vi "Sort 2D String Array - Preview Sorted Array.vi"(7 "Sorted Data Preview":string[][](table)) -> (8 "Output Array":string[][](array[string]), 10 "User Cancelled":bool)   [LabVIEW 2009]
doc: "Sort 2D String Array - Preview Sorted Array.vi\n\n<B>Description:</B>\n\nThis VI enables the user to preview the sorted array and accept or cancel the sort.\n\nThe user can press the Accept Sort button to accept the sorted array as displayed. If the Accept Sort button is pressed, the input array is passed to the Output Array terminal.\n\nThe user can press the Cancel Sort button to cancel the sort. If the Cancel Sort button is pressed, an empty array is passed to the Output Array terminal.\n\n<B>Usage:</B>\n\nWire all required inputs.\n\n<B>Inputs:</B>\n\nSorted Data Preview\n- This is the input 2D array of strings that will be previewed.\n\n<B>Outputs:</B>\n\nUser Cancelled\n- This output is set True if the user selects the cancel button.\n\nOutput Array\n- This is the Output Array. If the Accept Sort button is pressed, the input array is passed to the Output Array terminal.\n\nIf the Cancel Sort button is pressed, an empty array is passed to the Output Array terminal.\n\n<B>Developed by:</B>\n\nMark Ridgley\nmark.ridgley@logicpd.com"
panel:
  in  "Cancel Sort":bool
  in  "Accept Sort":bool
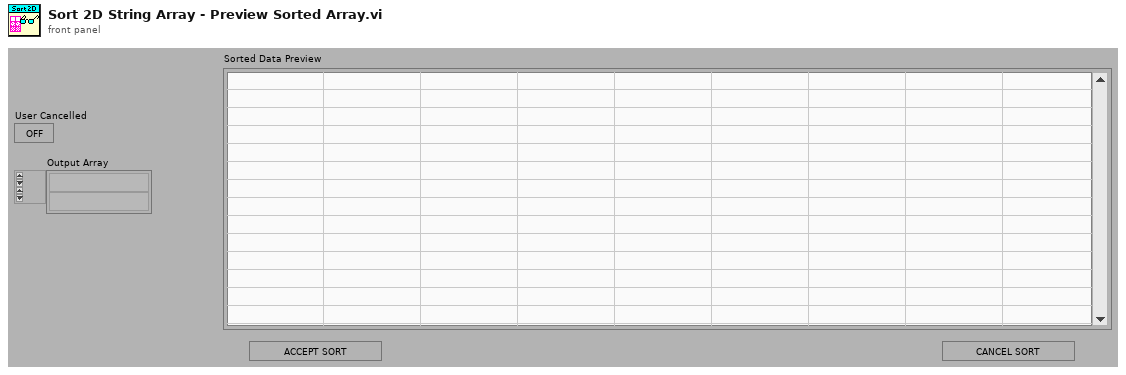
[diagram p1: front panel]
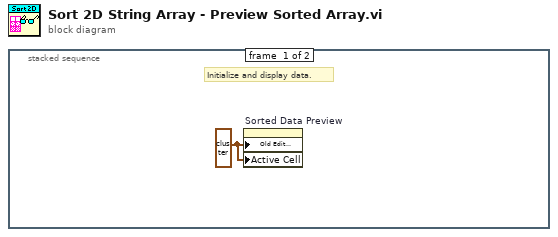
[diagram p0: block diagram]
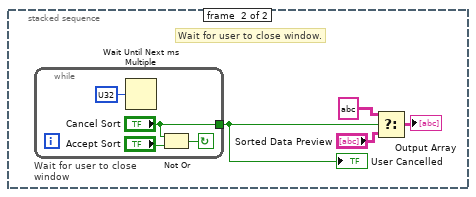
[diagram p2: hidden frame]
diagram:
  n1 = stacked-sequence {
    frame #0 {
      w1 = cluster{i32, i32} ? ("Write Attribute")
      # "Initialize and display data."
      n2 = property on="Sorted Data Preview" class="Tbl (strict)"("Old Edit Position"=w1, "Active Cell"=w1) -> ()  [unwired: 2 in, 2 out]
    }
    frame #1 {
      # "Wait for user to close window."
      n3 = while "Wait for user to close window" {
        tunnel: ["Cancel Sort"] -> w5
        stop <- w8 continue-if-true
        n4 = Wait Until Next ms Multiple(millisecond multiple=u32 ?) -> ()  [unwired: 1 out]
        n5 = Not Or(1:"Accept Sort", 2:"Cancel Sort") -> (0:w8:bool)
      }
      "User Cancelled" <- w5
      n6 = Select(t=string[][] ? ("Sorted Array"), s=w5, f="Sorted Data Preview") -> (s? t:f=→"Output Array":string[][])
    }
  }
